vi "AutoFeedForwardConversion.vi"(1 "Target Velocity (in/s)":dbl) -> (0 "Equivalent Joystick Command":dbl)   [LabVIEW 2019]
doc: "Converts the feed-forward path goal velocity from inches/sec to a the unitless drive command. This VI is intended for use with the FRC 4265 Autonomous Path Planner and the pure-pursuit algorithm. The input is in inches per second and the output is a unitless equivalent joystick command."
panel:
  in  "Maximum Robot Ground Speed (in/s)":dbl=197.0 format="%#_13g"
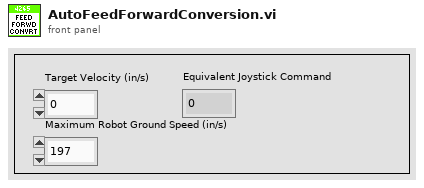
[diagram p1: front panel]
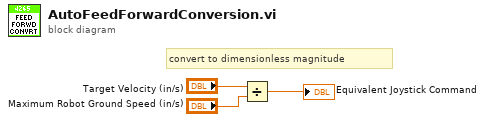
[diagram p0: block diagram]
diagram:
  # "convert to dimensionless magnitude"
  n1 = Divide(x="Target Velocity (in/s)", y="Maximum Robot Ground Speed (in/s)") -> (x/y=→"Equivalent Joystick Command":dbl)
